vi "uarv_grafici.vi"() -> ()   [LabVIEW 2023]
uses:
  <vilib>/Utility/miscctls.llb/LVForegroundBackgroundColorsTypeDef.ctl
  enum_typedef.ctl
panel:
  in  "STOP":bool
  in  "10D":bool
  in  "5D":bool
  out "STANJE":T1
  out "error out":errorcluster
  in  "error in (no error)":errorcluster
  in  "stop":bool
  in  "10D":bool
  in  "5D":bool
  out "STANJE":T1
  in  "Plot Area:Colors":T2
  in  "POKRENI":bool
  in  "Enum":enum16{"SINE", "COSINE"}(ring)
  out "Waveform Graph 5":dbl[](graph)
  out "Waveform Graph 4":dynamicdata(graph)
  out "Waveform Graph 3":dynamicdata(graph)
  out "Waveform Graph 2":waveform(dbl)[](graph)
  out "Waveform Graph":dbl[][](graph)
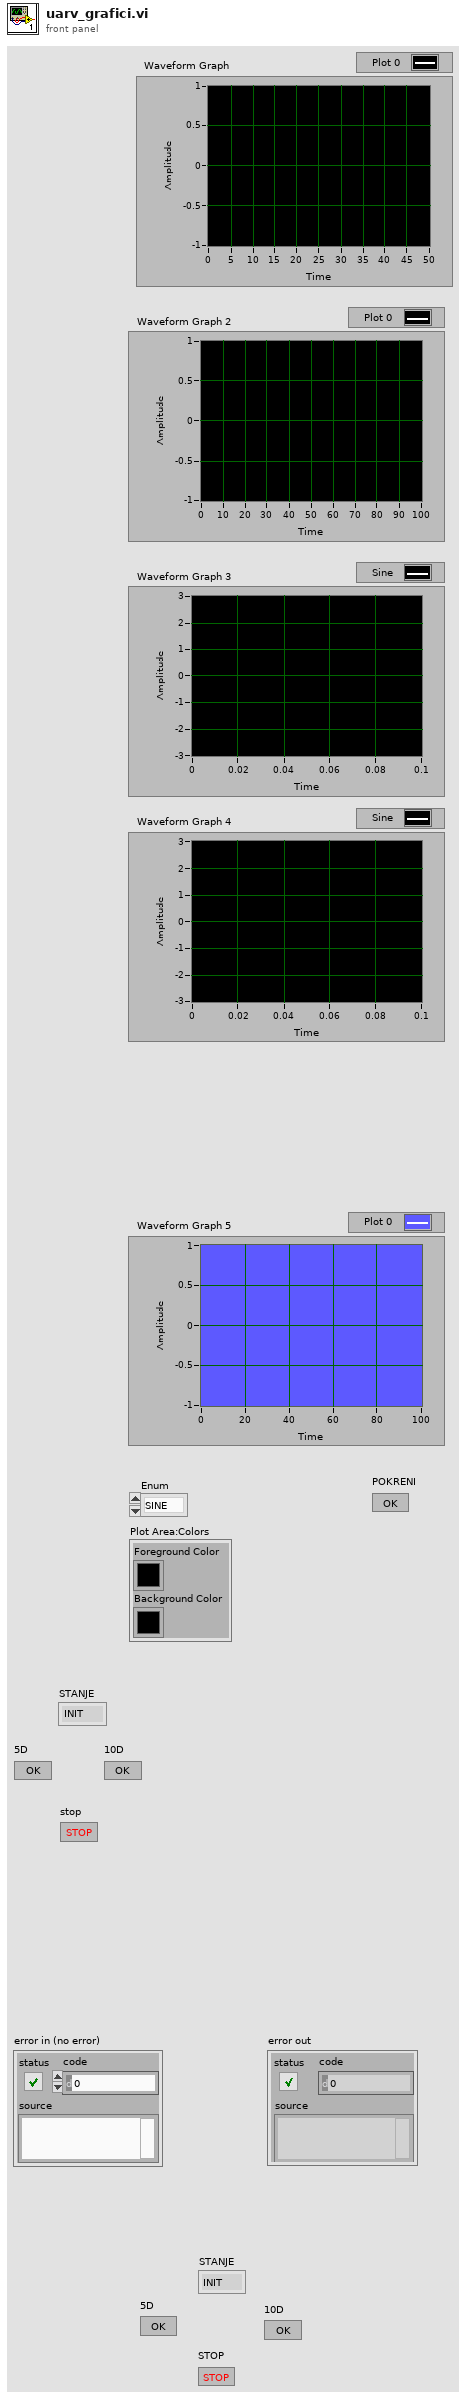
[diagram p1: front panel]
types:
  T1 = typedef "enum_typedef.ctl" = enum16{"INIT", "5D", "10D", "15D", "20D", "KUSUR"}
  T2 = typedef "LVForegroundBackgroundColorsTypeDef.ctl" = cluster{"Foreground Color":u32, "Background Color":u32}
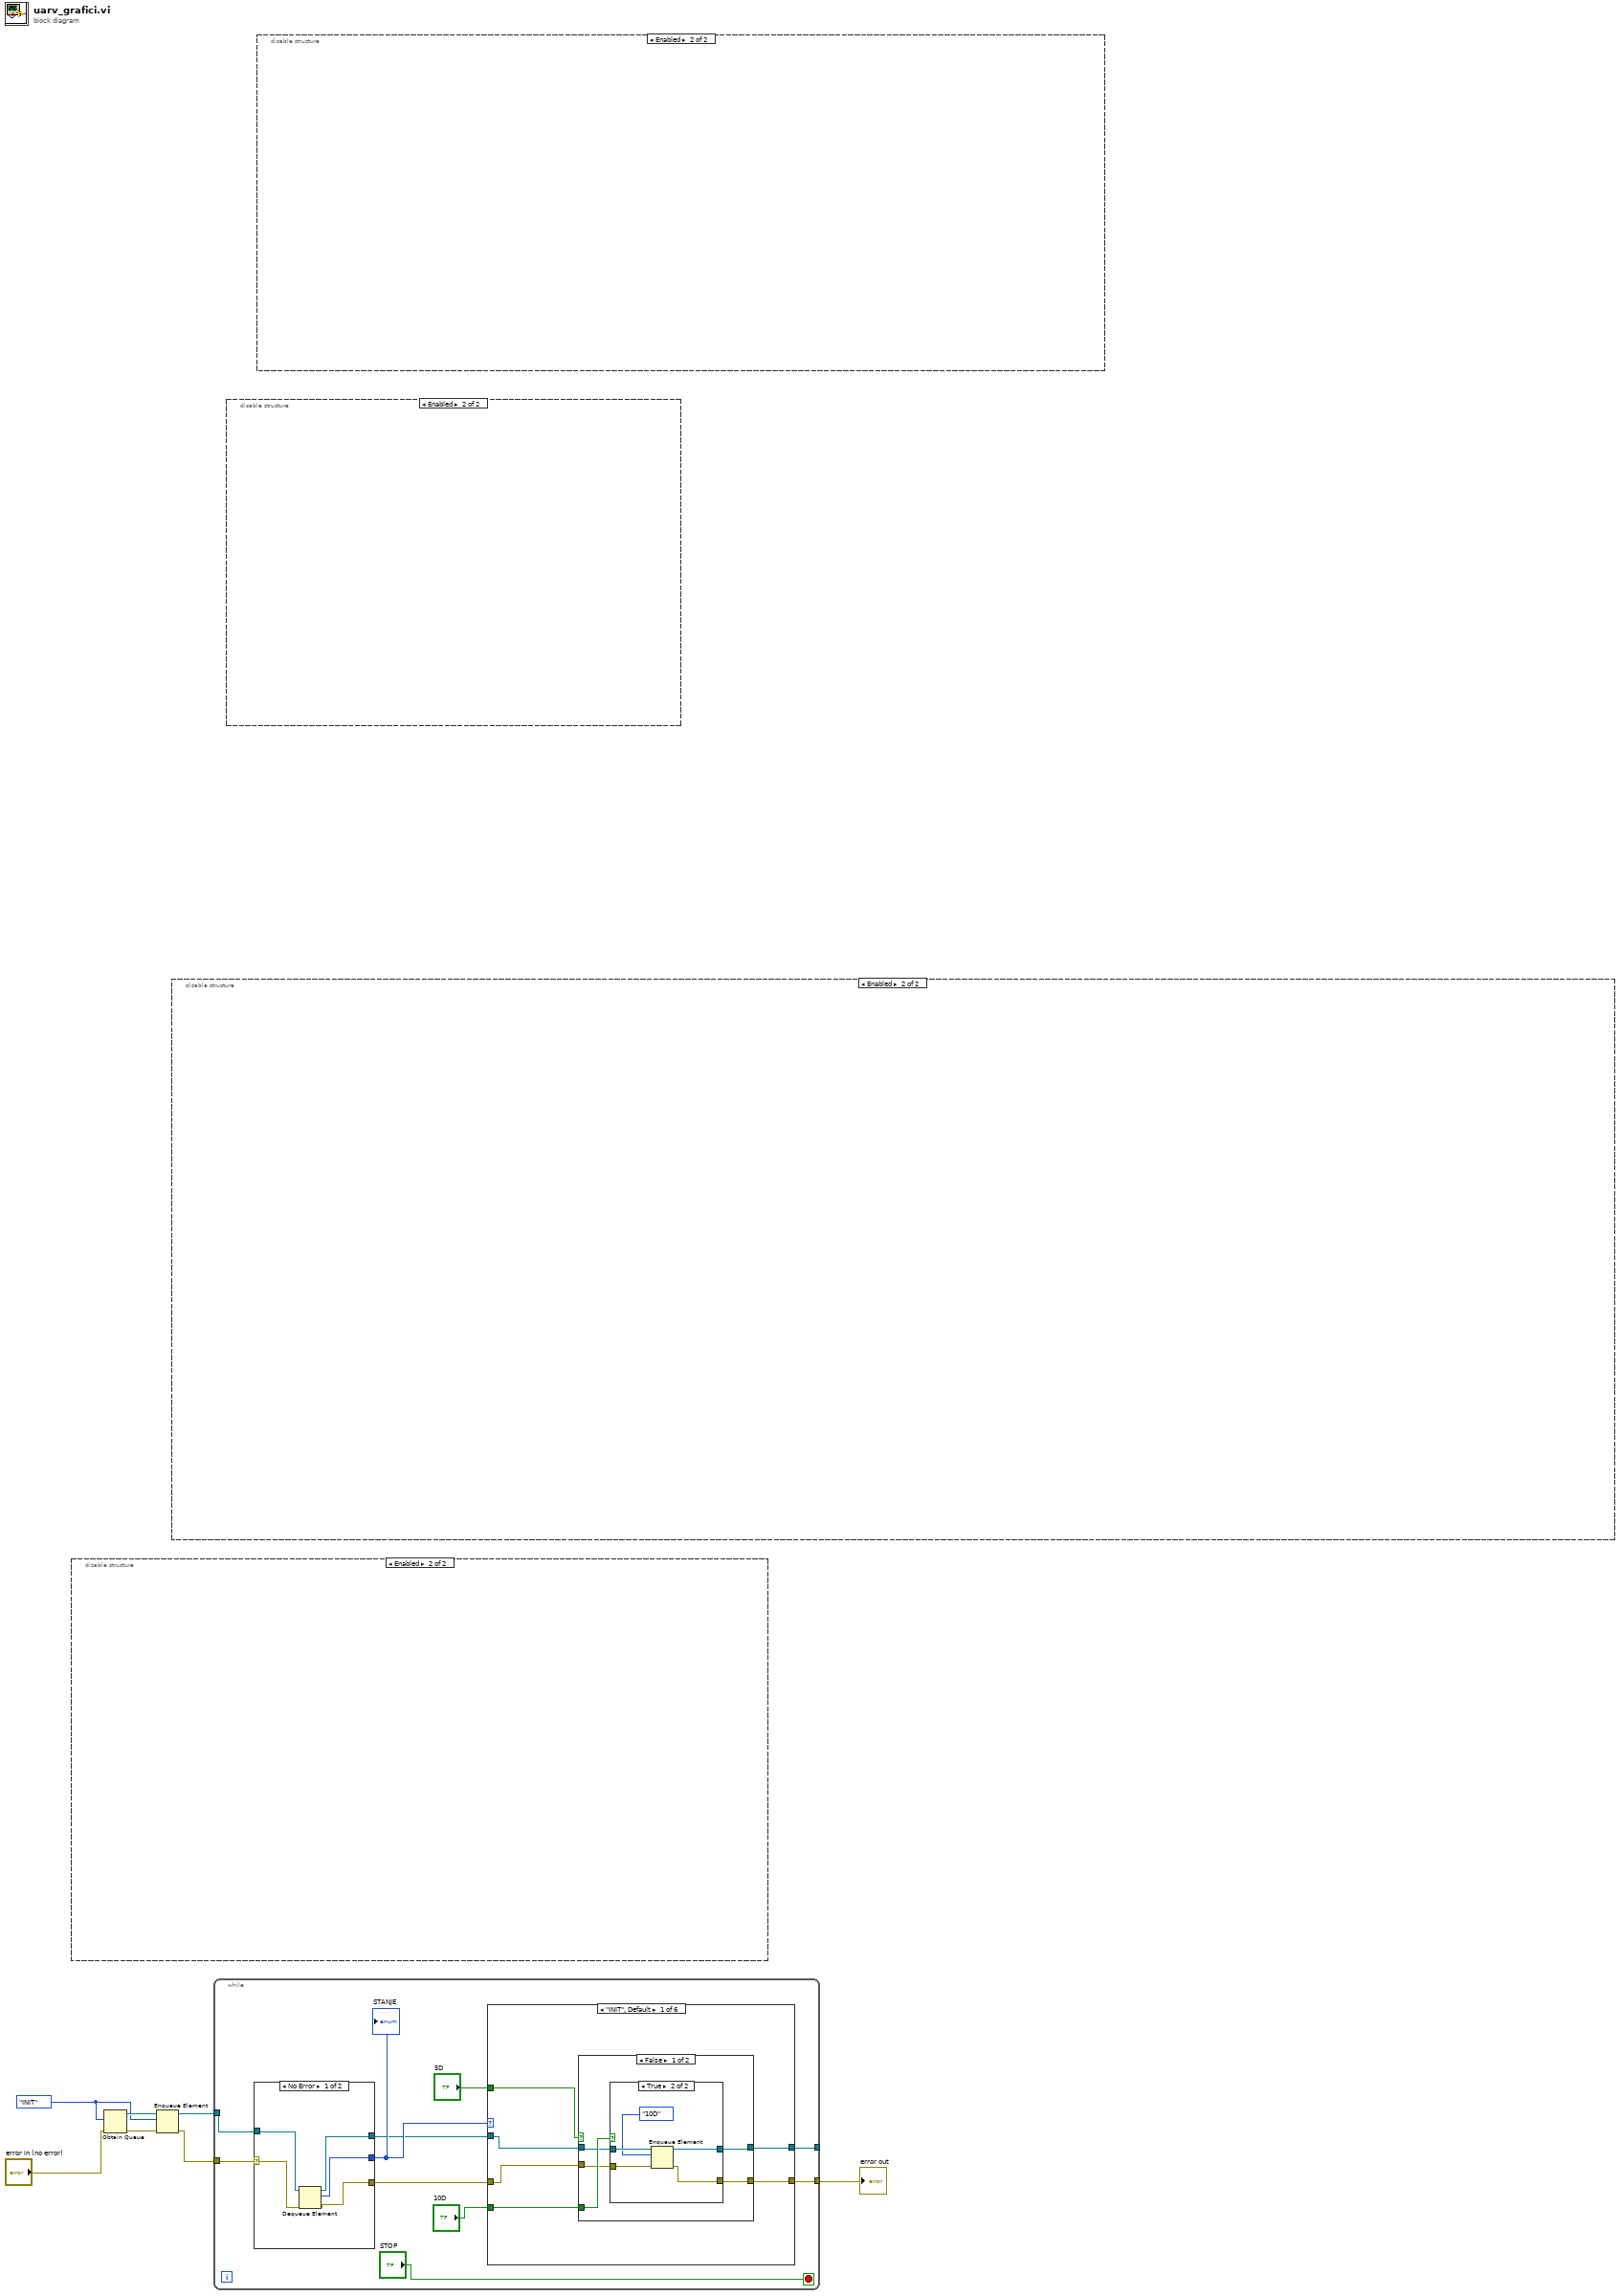
[diagram p0: block diagram]
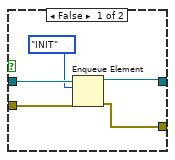
[diagram p2: hidden frame]
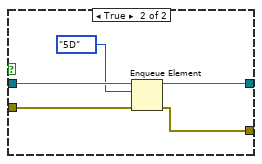
[diagram p3: hidden frame]
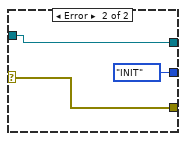
[diagram p9: hidden frame]
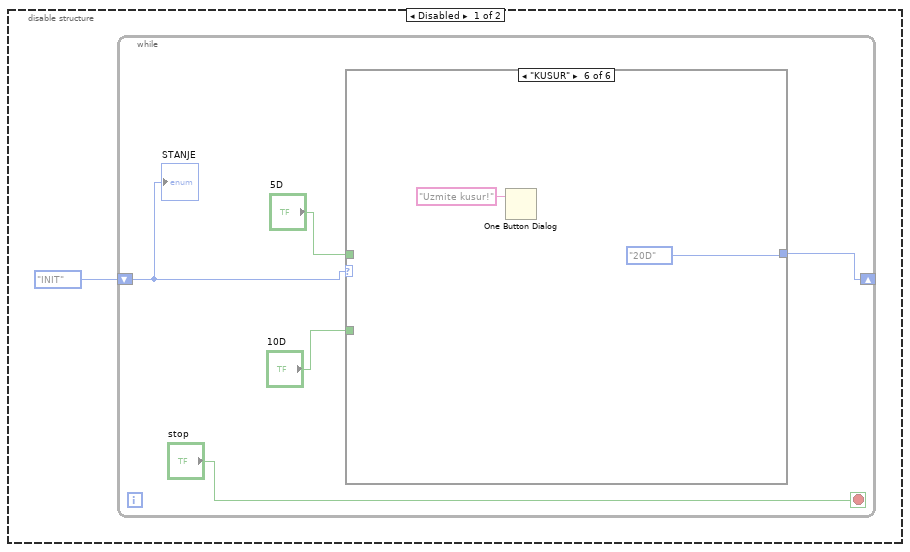
[diagram p10: hidden frame]
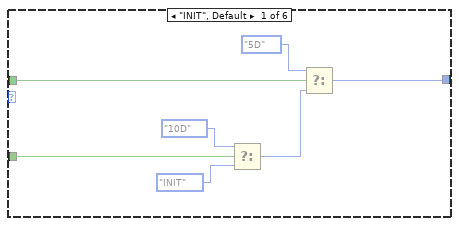
[diagram p11: hidden frame]
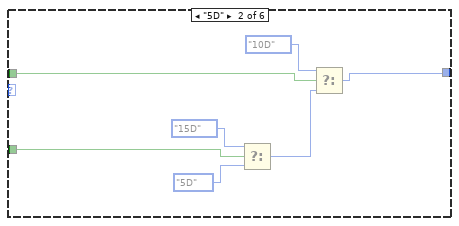
[diagram p12: hidden frame]
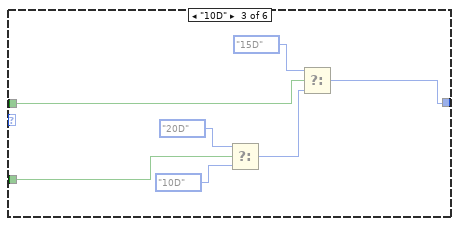
[diagram p13: hidden frame]
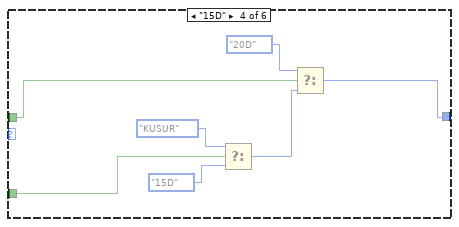
[diagram p14: hidden frame]
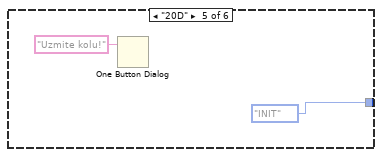
[diagram p15: hidden frame]
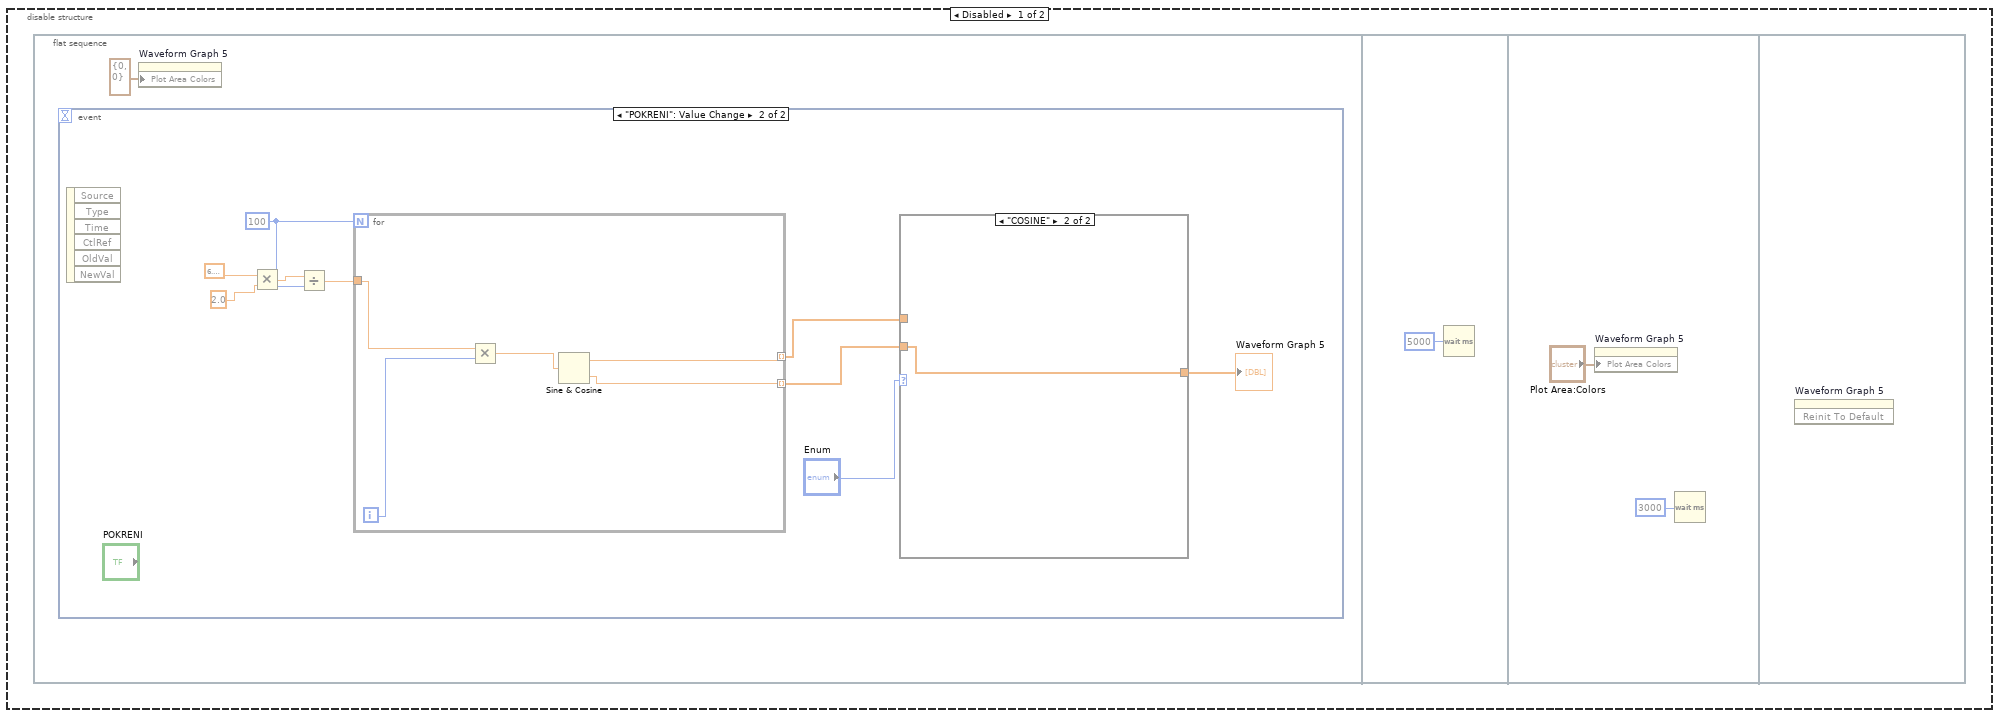
[diagram p16: hidden frame]
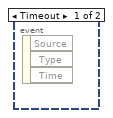
[diagram p17: hidden frame]
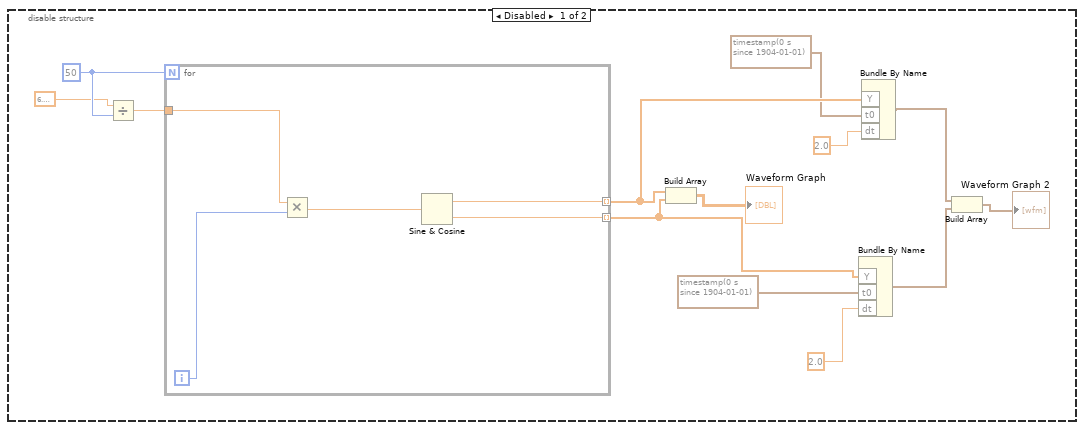
[diagram p19: hidden frame]
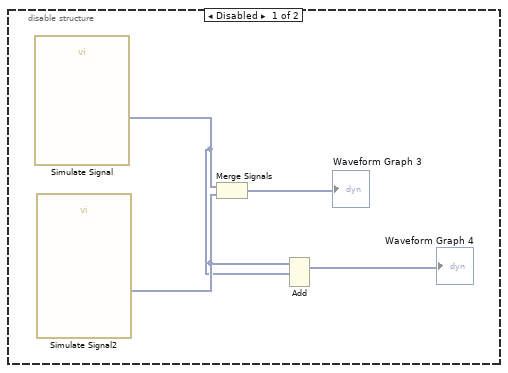
[diagram p20: hidden frame]
diagram:
  w2 = enum_typedef."INIT" ("Enum 2")
  n1 = disable-structure shown="Enabled" {
    frame Disabled {
      n2 = while {
        shift-right: [w12] -> _
        shift-left: enum_typedef."INIT" ("Enum 2") -> [w13]
        stop <- "stop" stop-if-true
        n3 = case shown="\"KUSUR\"" w13 {
          tunnel: [w16 w21 w28 w35 enum_typedef."INIT" ("Enum 2") enum_typedef."20D" ("Enum 2")] -> w12
          tunnel: "5D" -> [w15 w23 w29 w36 _ _]
          tunnel: "10D" -> [w14 w22 w31 w37 _ _]
          frame "INIT", Default {
            n4 = Select(t=enum_typedef."10D" ("Enum 2"), s=w14, f=enum_typedef."INIT") -> (s? t:f=w20:T1)
            n5 = Select(t=enum_typedef."5D", s=w15, f=w20) -> (s? t:f=w16:T1)
          }
          frame "5D" {
            n6 = Select(t=enum_typedef."15D" ("Enum 2"), s=w22, f=enum_typedef."5D") -> (s? t:f=w27:T1)
            n7 = Select(t=enum_typedef."10D", s=w23, f=w27) -> (s? t:f=w21:T1)
          }
          frame "10D" {
            n8 = Select(t=enum_typedef."20D" ("Enum 2"), s=w31, f=enum_typedef."10D") -> (s? t:f=w30:T1)
            n9 = Select(t=enum_typedef."15D", s=w29, f=w30) -> (s? t:f=w28:T1)
          }
          frame "15D" {
            n10 = Select(t=enum_typedef."KUSUR" ("Enum 2"), s=w37, f=enum_typedef."15D") -> (s? t:f=w41:T1)
            n11 = Select(t=enum_typedef."20D", s=w36, f=w41) -> (s? t:f=w35:T1)
          }
          frame "20D" {
            n12 = One Button Dialog(message="Uzmite kolu!") -> ()  [unwired: 1 in, 1 out]
          }
          frame "KUSUR" {
            n13 = One Button Dialog(message="Uzmite kusur!") -> ()  [unwired: 1 in, 1 out]
          }
        }
        "STANJE" <- w13
      }
    }
    frame Enabled {
    }
  }
  n14 = Obtain Queue(element data type=w2, error in (no error)="error in (no error)") -> (queue out=w7:refnum<queue>, error out=w6:errorcluster)  [unwired: 3 in, 1 out]
  n15 = Enqueue Element(queue=w7, element=w2, error in (no error)=w6) -> (queue out=w3:refnum<queue>, error out=w4:errorcluster)  [unwired: 1 in, 1 out]
  n16 = disable-structure shown="Enabled" {
    frame Disabled {
      n17 = flat-sequence {
        frame #0 {
          n18 = event shown="[1] \"POKRENI\": Value Change" {
            selector: _ -> [_ _]
            dyn-events: _ -> [_ _]
            timeout: _ -> [_ _]
            event Timeout {
              n19 = event-data() -> ()  [unwired: 1 in, 3 out]
            }
            event "POKRENI": Value Change {
              w49 = 100
              n20 = event-data() -> ()  [unwired: 1 in, 6 out]
              n21 = Multiply(x=6.283185307179586, y=2.0) -> (x*y=w50:dbl)
              n22 = Divide(x=w50, y=w49) -> (x/y=w51:dbl)
              n23 = for {
                N: w49 -> [_]
                tunnel: w51 -> [w61]
                tunnel: [w59] -> w53 mode=indexing
                tunnel: [w58] -> w54 mode=indexing
                i -> [w62]
                n24 = Multiply(x=w61, y=w62) -> (x*y=w60:dbl)
                n25 = Sine & Cosine(0:w60) -> (1:w59:dbl, 2:w58:dbl)
              }
              n26 = case shown="\"COSINE\"" "Enum" {
                tunnel: w53 -> [w56 _]
                tunnel: w54 -> [_ w57]
                tunnel: [w56 w57] -> w55
                frame "SINE", Default {
                }
                frame "COSINE" {
                }
              }
              "Waveform Graph 5" <- w55
            }
          }
          n27 = property on="Waveform Graph 5" class="WFGraph (strict)"("Plot Area Colors"=T2 {"Foreground Color"=0, "Background Color"=0} ("Plot Area:Colors")) -> ()  [unwired: 2 in, 2 out]
        }
        frame #1 {
          n28 = Wait (ms)(milliseconds to wait=u32 5000) -> ()  [unwired: 1 out]
        }
        frame #2 {
          n29 = property on="Waveform Graph 5" class="WFGraph (strict)"("Plot Area Colors"="Plot Area:Colors") -> ()  [unwired: 2 in, 2 out]
          n30 = Wait (ms)(milliseconds to wait=u32 3000) -> ()  [unwired: 1 out]
        }
        frame #3 {
          n31 = invoke on="Waveform Graph 5" class="WFGraph (strict)" method="Reinit To Default"() -> ()  [unwired: 3 in, 3 out]
        }
      }
    }
    frame Enabled {
    }
  }
  n32 = while {
    tunnel: w4 -> [w75]
    tunnel: w3 -> [w74]
    tunnel: [w68] -> w1
    tunnel: [w67] -> _
    stop <- "STOP" stop-if-true
    n33 = case shown="No Error" w75 {
      selector: w75 -> [w106 w107]
      tunnel: w74 -> [w104 w109]
      tunnel: [w105 w107] -> w72
      tunnel: [w103 enum_typedef."INIT" ("Enum 2")] -> w73
      tunnel: [w102 w109] -> w71
      frame No Error {
        n34 = Dequeue Element(queue=w104, error in (no error)=w106) -> (queue out=w102:refnum<queue>, element=w103:T1, error out=w105:errorcluster)  [unwired: 1 in, 1 out]
      }
      frame Error {
      }
    }
    "STANJE" <- w73
    n35 = case shown="\"INIT\", Default" w73 {
      tunnel: w72 -> [w79 _ _ _ _ _]
      tunnel: w71 -> [w80 _ _ _ _ _]
      tunnel: "5D" -> [w81 _ _ _ _ _]
      tunnel: [w78 _ _ _ _ _] -> w68
      tunnel: [w77 _ _ _ _ _] -> w67
      tunnel: "10D" -> [w76 _ _ _ _ _]
      frame "INIT", Default {
        n36 = case shown="False" w81 {
          tunnel: w80 -> [w83 w101]
          tunnel: w79 -> [w84 w100]
          tunnel: [w85 w99] -> w78
          tunnel: [w82 w98] -> w77
          tunnel: w76 -> [w86 _]
          frame False {
            n37 = case shown="True" w86 {
              tunnel: [w91 w96] -> w85
              tunnel: w84 -> [w88 w95]
              tunnel: w83 -> [w89 w94]
              tunnel: [w90 w93] -> w82
              frame False {
                n38 = Enqueue Element(queue=w89, element=enum_typedef."INIT", error in (no error)=w88) -> (queue out=w90:refnum<queue>, error out=w91:errorcluster)  [unwired: 1 in, 1 out]
              }
              frame True {
                n39 = Enqueue Element(queue=w94, element=enum_typedef."10D", error in (no error)=w95) -> (queue out=w93:refnum<queue>, error out=w96:errorcluster)  [unwired: 1 in, 1 out]
              }
            }
          }
          frame True {
            n40 = Enqueue Element(queue=w101, element=enum_typedef."5D", error in (no error)=w100) -> (queue out=w98:refnum<queue>, error out=w99:errorcluster)  [unwired: 1 in, 1 out]
          }
        }
      }
      frame "5D" {
      }
      frame "10D" {
      }
      frame "15D" {
      }
      frame "20D" {
      }
      frame "KUSUR" {
      }
    }
  }
  "error out" <- w1
  n41 = disable-structure shown="Enabled" {
    frame Disabled {
      n42 = call "Simulate Signal"() -> ("Sine"=w111:dynamicdata)  [unwired: 14 in, 1 out]
      n43 = call "Simulate Signal2"() -> ("Sine"=w112:dynamicdata)  [unwired: 14 in, 1 out]
      n44 = Merge Signals(w111, w112) -> (→"Waveform Graph 3":dynamicdata)
      n45 = Add(1:w111, 2:w112) -> (0:→"Waveform Graph 4":dynamicdata)  [unwired: 1 in, 1 out]
    }
    frame Enabled {
    }
  }
  n46 = disable-structure shown="Enabled" {
    frame Disabled {
      w126 = 50
      n47 = Divide(x=6.283185307179586, y=w126) -> (x/y=w124:dbl)
      n48 = for {
        N: w126 -> [_]
        tunnel: w124 -> [w130]
        tunnel: [w128] -> w119 mode=indexing
        tunnel: [w127] -> w120 mode=indexing
        i -> [w131]
        n49 = Multiply(x=w130, y=w131) -> (x*y=w129:dbl)
        n50 = Sine & Cosine(0:w129) -> (1:w128:dbl, 2:w127:dbl)
      }
      n51 = Build Array(w119, w120) -> (→"Waveform Graph":dbl[][])
      n52 = Bundle By Name("Y"=w120, "t0"=timestamp(0 s since 1904-01-01), "dt"=2.0) -> (w114:waveform(dbl))  [unwired: 1 in]
      n53 = Bundle By Name("Y"=w119, "t0"=timestamp(0 s since 1904-01-01), "dt"=2.0) -> (w115:waveform(dbl))  [unwired: 1 in]
      n54 = Build Array(w115, w114) -> (→"Waveform Graph 2":waveform(dbl)[])
    }
    frame Enabled {
    }
  }
